vi "Close Ref.vi"(8 "error in (no error)":errorcluster, 11 "AIT 429 in":refnum<class "AIT 429.lvclass">) -> (0 "error out":errorcluster, 3 "AIT 429 out":refnum<class "AIT 429.lvclass">)   [LabVIEW 2016, in "ARINC.lvlib" / "AIT 429.lvclass"]
uses:
  AIT 429.lvclass
  AIT 429.lvclass/AIT 429.ctl
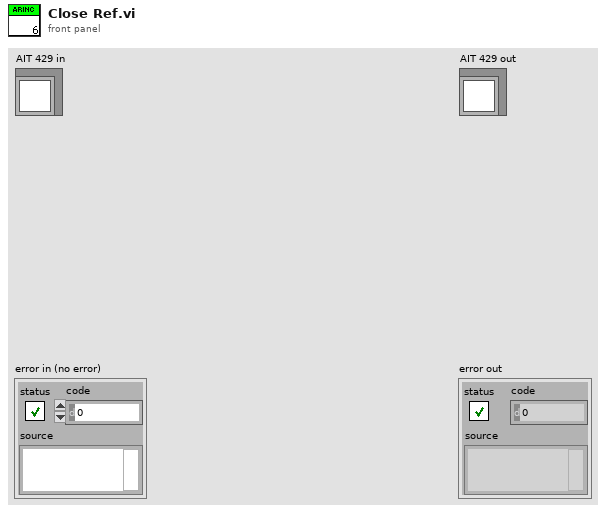
[diagram p1: front panel]
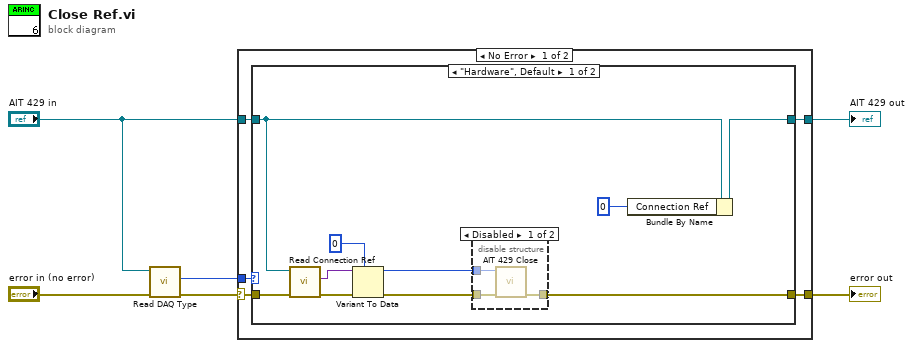
[diagram p0: block diagram]
diagram:
  n1 = call-dynamic "Read DAQ Type.vi"("error in (no error)"="error in (no error)", "AIT 429 in"="AIT 429 in") -> ("error out"=w5:errorcluster, "DAQ Type"=w4:enum16{"Hardware", "Simulation"})  [unwired: 7 in, 1 out]
  n2 = case shown="No Error" w5 {
    selector: w5 -> [w10 w27]
    tunnel: "AIT 429 in" -> [w9 w28]
    tunnel: w4 -> [w11 _]
    tunnel: [w8 w28] -> w2
    tunnel: [w7 w27] -> w1
    frame No Error {
      n3 = case shown="\"Hardware\", Default" w11 {
        tunnel: w10 -> [w21 w25]
        tunnel: w9 -> [w15 w26]
        tunnel: [w13 w26] -> w8
        tunnel: [w14 w25] -> w7
        frame "Hardware", Default {
          n4 = call-dynamic "Read Connection Ref.vi"("error in (no error)"=w21, "AIT 429 in"=w15) -> ("error out"=w20:errorcluster, "Connection Ref"=w18:variant)  [unwired: 7 in, 1 out]
          n5 = Variant To Data(error in=w20, type=u32 0 ("board handle"), Variant=w18) -> (data=w16:u32, error out=w19:errorcluster)
          n6 = disable-structure shown="Disabled" {
            disable-tunnel: w19 -> [w24 _]
            disable-tunnel: w16 -> [w23 _]
            disable-tunnel: [w22 _] -> w14
            frame Disabled {
              n7 = call <instrlib>:"AIT 429 Close.vi"("error in (no error)"=w24, "board handle"=w23) -> ("error out"=w22:errorcluster)  [unwired: 9 in]
            }
            frame Enabled {
            }
          }
          n8 = Bundle By Name(cluster=w15, "Connection Ref"=u32 0 ("board handle")) -> (w13:refnum<class "AIT 429.lvclass">)
        }
        frame "Simulation" {
        }
      }
    }
    frame Error {
    }
  }
  "error out" <- w1
  "AIT 429 out" <- w2
